vi "WriteFileContent.vi"(8 "error in":errorcluster, 9 "delimited string":string, 11 "File path in":path) -> (0 "error out":errorcluster, 3 "File path out":path)   [LabVIEW 2021]
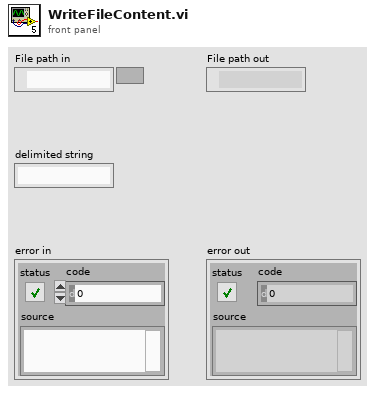
[diagram p1: front panel]
types:
  T1 = enum16{"open", "replace", "create", "open or create", "replace or create", "replace or create with confirmation"}
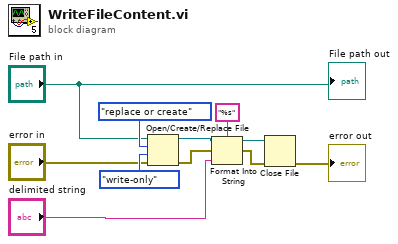
[diagram p0: block diagram]
diagram:
  n1 = Open/Create/Replace File(file path (use dialog)="File path in", error in="error in", operation (0:open)=T1."replace or create", access (0:read/write)=enum16{"read/write", "read-only", "write-only"}."write-only") -> (refnum out=w6:refnum<file>, error out=w7:errorcluster)  [unwired: 2 in, 1 out]
  n2 = Format Into String(format string="%s", initial string=w6, error in=w7, "delimited string") -> (resulting string=w10:refnum<file>, error out=w9:errorcluster)
  n3 = Close File(refnum=w10, error in=w9) -> (error out=→"error out":errorcluster)  [unwired: 1 out]
  "File path out" <- "File path in"
